vi "BB_LoadSettings.vi"(8 "Section":string="LowCamera", 10 "Array":cluster{string[]}[](array[cluster]), 11 "All User Path":path) -> (2 "Cluster":cluster{"value":i32, "value":i32, "index":i32}, 3 "Refnum out":T1)   [LabVIEW 2012]
uses:
  <vilib>/Utility/config.llb/Config Data RefNum.ctl
  <vilib>/Utility/config.llb/Read Key (String).vi
  <vilib>/Utility/config.llb/Read Key (I32).vi
  <vilib>/Utility/config.llb/NI_LVConfig.lvlib
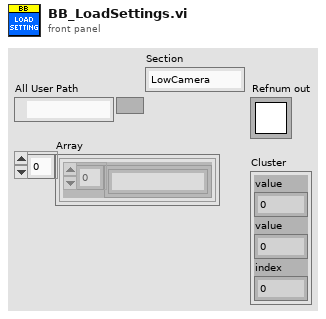
[diagram p1: front panel]
types:
  T1 = typedef "NI_LVConfig.lvlib/Config Data RefNum.ctl" = refnum<k1>
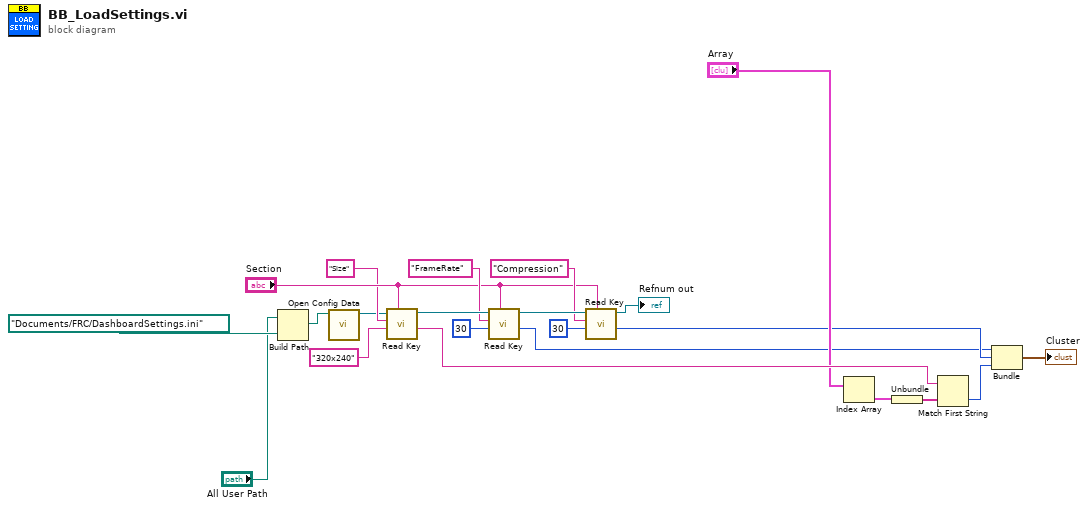
[diagram p0: block diagram]
diagram:
  n1 = Build Path(base path="All User Path", name or relative path=path "Documents/FRC/DashboardSettings.ini") -> (appended path=w2:path)
  n2 = call <vilib>:"Open Config Data.vi"("configuration file path"=w2) -> ("refnum"=w3:T1)  [unwired: 8 in, 2 out]
  n3 = call-poly <vilib>:"Read Key.vi"("section"="Section", "default value"="320x240", "key"="Size", "refnum"=w3) -> ("value"=w16:string, "refnum out"=w19:T1)  [unwired: 2 in, 4 out]
  n4 = call-poly <vilib>:"Read Key.vi"("section"="Section", "default value"=30, "key"="FrameRate", "refnum"=w19) -> ("value"=w11:i32, "refnum out"=w20:T1)  [unwired: 1 in, 5 out]
  n5 = call-poly <vilib>:"Read Key.vi"("section"="Section", "default value"=30, "key"="Compression", "refnum"=w20) -> ("value"=w12:i32, "refnum out"=→"Refnum out":T1)  [unwired: 1 in, 5 out]
  n6 = Index Array(array="Array") -> (element=w13:cluster{string[]})  [unwired: 1 in]
  n7 = Unbundle(w13) -> (w15:string[])
  n8 = Match First String(2:w15, 3:w16) -> (0:w17:i32)  [unwired: 1 out]
  n9 = Bundle("value"=w11, "value"=w12, "index"=w17) -> (→"Cluster":cluster{"value":i32, "value":i32, "index":i32})  [unwired: 1 out]
